vi "SelMeasFunc.vi"(8 "ErrorIn(No Error)":errorcluster caption="entrée d'erreur (pas d'erreur)", 9 "Active MeasPar":bool[](array[boolean]), 10 "ScanHeaderIn":i32[](array[numeric]), 11 "MeasIndexIn":i32[](array[numeric])) -> (0 "sortie d'erreur":errorcluster, 2 "ScanHeaderOut":i32[](array[numeric]), 3 "MeasIndexOut":i32[](array[numeric]))   [LabVIEW 2019]
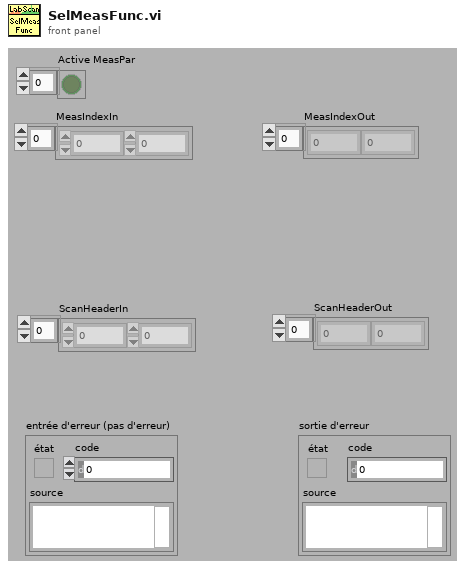
[diagram p1: front panel]
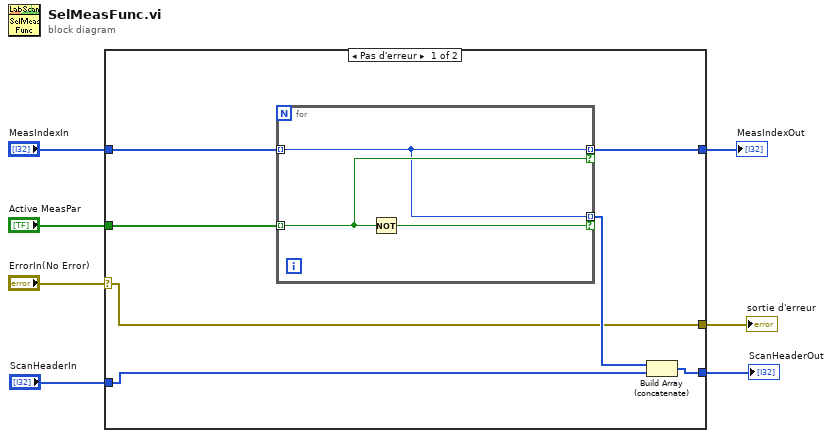
[diagram p0: block diagram]
diagram:
  n1 = case shown="Pas d'erreur" "ErrorIn(No Error)" {
    selector: "ErrorIn(No Error)" -> [w8 w19]
    tunnel: [w8 w19] -> w6
    tunnel: "MeasIndexIn" -> [w12 _]
    tunnel: "Active MeasPar" -> [w14 _]
    tunnel: [w13 _] -> w3
    tunnel: "ScanHeaderIn" -> [w10 w18]
    tunnel: [w9 w18] -> w1
    frame No Error {
      n2 = for {
        tunnel: [w16] -> w13 mode=indexing if=w17
        tunnel: w14 -> [w17] mode=indexing
        tunnel: w12 -> [w16] mode=indexing
        tunnel: [w16] -> w11 mode=indexing if=w15
        n3 = Not(x=w17) -> (.not. x?=w15:bool)
      }
      n4 = Build Array (concatenate)(w11, w10) -> (w9:i32[])
    }
    frame Error {
    }
  }
  "sortie d'erreur" <- w6
  "MeasIndexOut" <- w3
  "ScanHeaderOut" <- w1
